vi "Stop Core.vi"(10 "final error code":i32, 11 "AsmTestMachine in":refnum<class "AsmTestMachine.lvclass">) -> (3 "AsmTestMachine out":refnum<class "AsmTestMachine.lvclass">)   [LabVIEW 2021, in "AsmTestMachine.lvlib" / "AsmTestMachine.lvclass"]
doc: "(<B>Filename</B>: Actor Framework.lvlib:Actor.lvclass:Stop Core.vi)\n\nDefines what the actor does before it stops. Use the <B>final error code</B> input to determine whether the actor shut down in response to an error.\n\nBy default, this method passes the Stop message along to all auto-stop nested actors. A descendant class may override this method to define additional behavior, such as shutting down any processes the actor initiated in its override of the Actor Core method."
uses:
  AsmTestMachine.lvclass
  AsmTestMachine.lvclass/AsmTestMachine.ctl
  Source/ActorStateMachine/ActorStateMachine/ActorStateMachine.lvclass
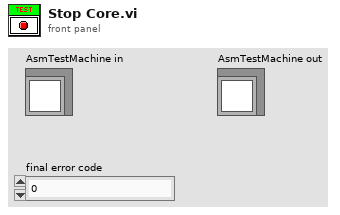
[diagram p1: front panel]
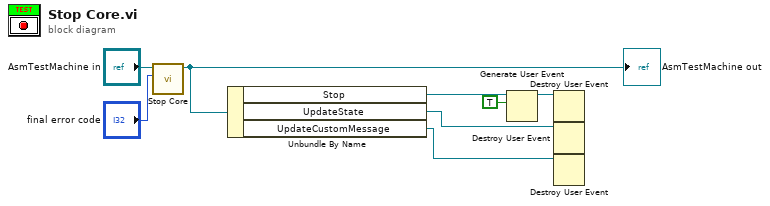
[diagram p0: block diagram]
diagram:
  n1 = call-parent "Stop Core.vi"("final error code"="final error code", "ActorStateMachine in"="AsmTestMachine in") -> ("ActorStateMachine out"=w6:refnum<class "AsmTestMachine.lvclass">)  [unwired: 9 in]
  "AsmTestMachine out" <- w6
  n2 = Unbundle By Name(w6) -> ("Stop"=w5:refnum<user-event>, "UpdateState"=w2:refnum<user-event>, "UpdateCustomMessage"=w1:refnum<user-event>)
  n3 = Generate User Event(user event=w5, event data cluster=TRUE ("event data")) -> (user event out=w3:refnum<user-event>)  [unwired: 2 in, 1 out]
  n4 = Destroy User Event(user event=w3) -> ()  [unwired: 1 in, 1 out]
  n5 = Destroy User Event(user event=w2) -> ()  [unwired: 1 in, 1 out]
  n6 = Destroy User Event(user event=w1) -> ()  [unwired: 1 in, 1 out]
